vi "DAQ_E_mIO_DIO.write word.vi"(0 "i ref in":refnum<vi>, 2 "word":u32, 3 "ms timeout (10000)":i32=10000, 4 "wordIndex":i32, 5 "error in (no error)":errorcluster) -> (14 "i ref out":refnum<vi>, 17 "timed out":bool, 19 "error out":errorcluster)   [LabVIEW 2014, in "DAQ_E_mIO_DIO.lvlib"]
doc: "Write a 8 bit word to the digital output port.\n\nLicense Agreement for this software:\n\nCopyright (C)\nGesellschaft für Schwerionenforschung, GSI\nPlanckstr. 1\n64291 Darmstadt\nGermany\n\nContact: D.Beck@gsi.de \n\nThis program is free software; you can redistribute it and/or modify it under the terms of the GNU General Public License as published by the Free Software Foundation; either version 2 of the license, or (at your option) any later version.\n\nThis program is distributed in the hope that it will be useful, but WITHOUT ANY WARRANTY; without even the implied warranty of MERCHANTABILITY or FITNESS FOR A PARTICULAR PURPOSE. See the GNU General License for more details (http://www.gnu.org).\n\nGesellschaft für Schwerionenforschung, GSI\nPlanckstr. 1, 64291 Darmstadt, Germany\nFor all questions and ideas contact: M.Richter@gsi.de, H.Brand@gsi.de or D.Beck@gsi.de.\nLast update: 17-JUN-2004"
uses:
  DAQ_E_mIO_DIO.lvlib
  CSCore/CSSystem/CoreDefs/CoreDefs.error_type.ctl
  CSApplicationBaseClasses/DigiIOBase/DigiIOBase.directionType.ctl
  CSApplicationBaseClasses/DigiIOBase/DigiIOBase.serviceType.ctl
  lib.lib/UtilityLib/UtilityLib.valueStatus.ctl
  <vilib>/DAQmx/write.llb/DAQmx Write (Digital 1D Bool 1Chan 1Samp).vi
  CSCore/CSSystem/CoreLib/CoreLib.lvlib
  CSApplicationBaseClasses/DigiIOBase/DigiIOBase.lvlib
  lib.lib/UtilityLib/UtilityLib.lvlib
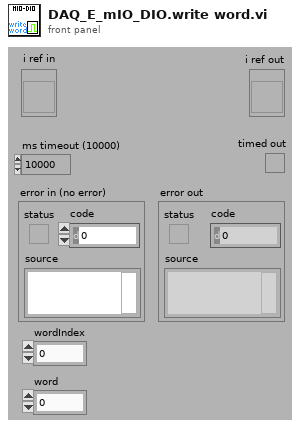
[diagram p1: front panel]
types:
  T1 = typedef "CoreDefs.error_type.ctl" = enum16{"no error", "can't load process", "can't unload process", "process does not exist", "can't install process", "can't remove process", "unknown function", "time out", "can't execute function", "duplicate queue name", "super not found", "caller queue invalid", "can't ping process", "unknown error", "VISA Error", "VISA timeout", "GPIB timeout", "GPIB error", "communication error", "data type mismatch", "can't read data from OPC server", "can't write data to OPC server", "OET error", "function not implemented", "process already exists", "invalid Shared Variable name", "error writing Shared Variable", "error reading Shared Variable", "invalid client name", "corrupt database", "unknown class", "call not authorized", "parameter out of range", "OET timeout: can't get data to modify", "invalid queue name", "requested operation incompatible with current state", "event undefined", "event disabled", "state undefined", "caller is not a friend", "EventBuilder: bad eventID", "EventBuilder: no DAQ devices", "a thread must not stop itself", "UNUSED ELEMENT4", "DiscArchiver: eventData incomplete", "DiscArchiver: eventData does not belong to run", "DiscArchiver: can't open file", "DiscArchiver: can't write to file", "DiscArchiver: available disc space low", "can't acquire semaphore", "error reading data from database", "notifier object is not existing", "can't register process", "can't unregister process", "illegal event type", "object disabled", "object already exists", "can't change state", "Instrument not found", "no connection to remote node", "invalid reference", "N/A", "UNUSED ELEMENT 1", "element not found", "illegal TCP/IP connection detected", "object does not exist", "invalid access ID", "unknown CS system", "invalid privilige", "unsupported data type", "unsupported server type", "IO server already exists", "Shared Variable already exists"}
  T2 = typedef "UtilityLib.lvlib/UtilityLib.valueStatus.ctl" = enum16{"no info available", "stand by/off", "on", "warning", "alarm/malfunction", "not implemented", "user action required", "important information", "system default", "control default", "indicator default", "button default"}
  T3 = typedef "DigiIOBase.lvlib/DigiIOBase.serviceType.ctl" = enum16{"bit", "word"}
  T4 = typedef "DigiIOBase.lvlib/DigiIOBase.directionType.ctl" = enum16{"unknown", "update actual value", "update nominal value", "update both"}
  T5 = typedef "DAQ_E_mIO_DIO.lvlib/DAQ_E_mIO_DIO.i attribute.ctl" = cluster{"DOutChannel":refnum<k21>, "DInChannel":refnum<k21>, "nOfBitsIn":i32, "nOfBitsOut":i32}
  T6 = typedef "DigiIOBase.lvlib/DigiIOBase.i attribute.ctl" = cluster{"logicalName":string[], "physicalName":string[], "logicalNameID":i32, "physicalNameID":i32, "nofBits":i32, "nofBitsID":i32, "nofWords":i32, "nofWordsID":i32, "nomValues":T7, "actValues":T7}
  T7 = typedef "DigiIOBase.lvlib/DigiIOBase.parameters.ctl" = cluster{"high":bool[], "serviceIDs":cluster{"highID":i32}}
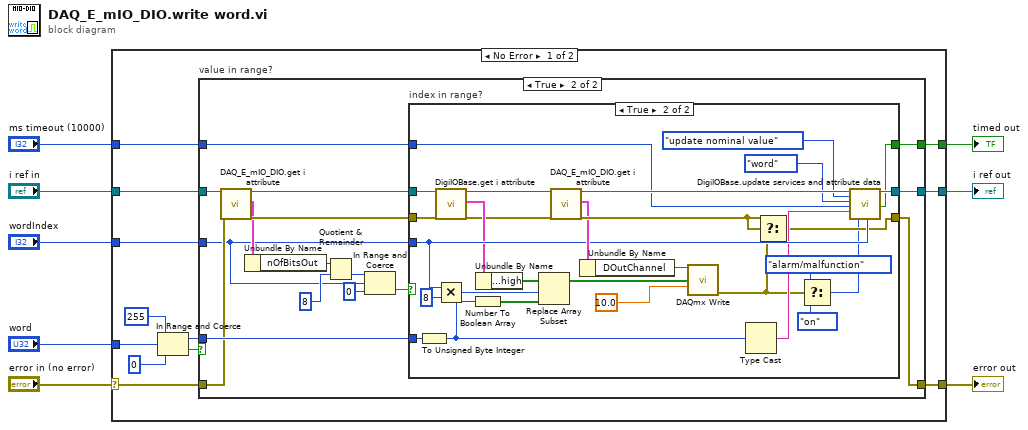
[diagram p0: block diagram]
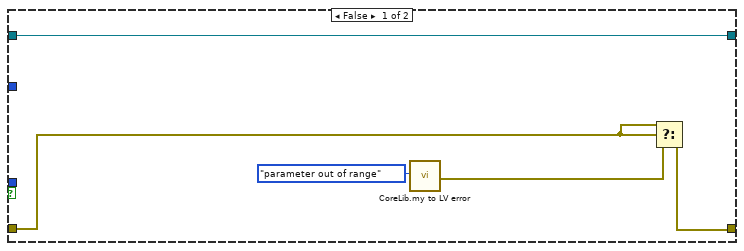
[diagram p2: hidden frame]
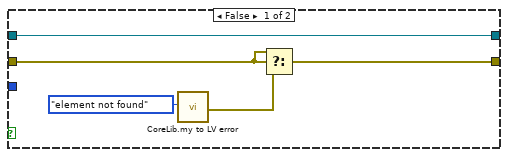
[diagram p3: hidden frame]
diagram:
  n1 = case shown="No Error" "error in (no error)" {
    selector: "error in (no error)" -> [w11 w76]
    tunnel: "i ref in" -> [w20 w77]
    tunnel: "ms timeout (10000)" -> [w19 _]
    tunnel: [w18 w77] -> w6
    tunnel: [w17 w76] -> w5
    tunnel: "word" -> [w15 _]
    tunnel: "wordIndex" -> [w10 _]
    tunnel: [w9 _] -> w1
    frame No Error {
      n2 = In Range and Coerce(upper limit=u32 255, x=w15, lower limit=u32 0) -> (coerced(x)=w14:u32, In Range?=w16:bool)
      n3 = case "value in range?" shown="True" w16 {
        tunnel: w20 -> [w25 w38]
        tunnel: w11 -> [w23 w37]
        tunnel: w19 -> [_ w34]
        tunnel: [w25 w41] -> w18
        tunnel: [w24 w39] -> w17
        tunnel: w14 -> [_ w40]
        tunnel: w10 -> [_ w28]
        tunnel: [_ w33] -> w9
        frame False {
          n4 = call "CoreLib.my to LV error.vi"("ErrorTypes"=CoreDefs.error_type."parameter out of range") -> ("myErrorCluster"=w22:errorcluster)  [unwired: 17 in, 1 out]
          n5 = Select(t=w23, s=w23, f=w22) -> (s? t:f=w24:errorcluster)
        }
        frame True {
          n6 = call "DAQ_E_mIO_DIO.get i attribute.vi"("i ref in"=w38, "error in (no error)"=w37) -> ("i ref out"=w36:refnum<vi>, "i attribute"=w32:T5, "error out"=w35:errorcluster)  [unwired: 15 in]
          n7 = Unbundle By Name(w32) -> ("nOfBitsOut"=w31:i32)
          n8 = Quotient & Remainder(x=w31, y=8) -> (floor(x/y)=w29:i32)  [unwired: 1 out]
          n9 = In Range and Coerce(upper limit=w29, x=w28, lower limit=0) -> (In Range?=w26:bool)  [unwired: 1 out]
          n10 = case "index in range?" shown="True" w26 {
            tunnel: w36 -> [w46 w60]
            tunnel: [w46 w69] -> w41
            tunnel: w40 -> [_ w64]
            tunnel: [w45 w52] -> w39
            tunnel: w35 -> [w44 w59]
            tunnel: w28 -> [_ w66]
            tunnel: w34 -> [_ w65]
            tunnel: [_ w62] -> w33
            frame False {
              n11 = call "CoreLib.my to LV error.vi"("ErrorTypes"=CoreDefs.error_type."element not found") -> ("myErrorCluster"=w43:errorcluster)  [unwired: 17 in, 1 out]
              n12 = Select(t=w44, s=w44, f=w43) -> (s? t:f=w45:errorcluster)
            }
            frame True {
              n13 = To Unsigned Byte Integer(number=w64) -> (unsigned 8bit integer=w61:u8)
              n14 = call "DigiIOBase.get i attribute.vi"("i ref in"=w60, "error in (no error)"=w59) -> ("i ref out"=w53:refnum<vi>, "i attribute"=w58:T6, "error out"=w51:errorcluster)  [unwired: 15 in]
              n15 = Multiply(x=w66, y=8) -> (x*y=w56:i32)
              n16 = Number To Boolean Array(number=w61) -> (Boolean array=w55:bool[])
              n17 = Unbundle By Name(w58) -> ("nomValues.high"=w57:bool[])
              n18 = Replace Array Subset(array=w57, new element=w55, index=w56) -> (w54:bool[])
              n19 = call "DAQ_E_mIO_DIO.get i attribute.vi"("i ref in"=w53, "error in (no error)"=w51) -> ("i ref out"=w70:refnum<vi>, "i attribute"=w74:T5, "error out"=w75:errorcluster)  [unwired: 15 in]
              n20 = Unbundle By Name(w74) -> ("DOutChannel"=w73:refnum<k21>)
              n21 = call-poly <vilib>:"DAQmx Write.vi"("task/channels in"=w73, "data"=w54, "timeout"=10.0) -> ("error out"=w50:errorcluster)  [unwired: 10 in, 2 out]
              n22 = Type Cast(x=w61) -> (*(type *) &x=w63:string)  [unwired: 1 in]
              n23 = Select(t=w75, s=w75, f=w50) -> (s? t:f=w52:errorcluster)
              n24 = Select(t=UtilityLib.valueStatus."alarm/malfunction" ("f"), s=w50, f=UtilityLib.valueStatus."on" ("quality")) -> (s? t:f=w49:T2)
              n25 = call "DigiIOBase.update services and attribute data.vi"("i ref in"=w70, "direction"=DigiIOBase.directionType."update nominal value", "service"=DigiIOBase.serviceType."word", "ms timeout (10000)"=w65, "value"=w63, "quality"=w49, "index"=w66) -> ("i ref out"=w69:refnum<vi>, "timed out"=w62:bool)  [unwired: 10 in, 1 out]
            }
          }
        }
      }
    }
    frame Error {
    }
  }
  "error out" <- w5
  "i ref out" <- w6
  "timed out" <- w1
